vi "Line Prototype 1.2.vi"() -> ()   [LabVIEW 2009]
uses:
  <vilib>/vision/Image Controls.llb/IMAQ Image.ctl
  <vilib>/Analysis/3filter.llb/Filter Passband Type.ctl
  <vilib>/Analysis/3filter.llb/Butterworth Filter (DBL).vi
  <vilib>/vision/NI_Vision_Development_Module.lvlib
  <vilib>/Analysis/NI_AALBase.lvlib
panel:
  in  "low  2":dbl=0.12500000000000006 format="%0.4f"
  in  "high 2":dbl=60.0 format="%0.2f"
  in  "sampling 2":dbl=1.0 format="%0.2f"
  out "LED BLUE":bool
  out "Waveform RED 2":dbl[](graph)
  in  "playtime":dbl=10.0
  out "Frame Number":i32
  in  "Frame Start":i32=2100
  out "LED RED":bool
  in  "low":dbl=0.12500000000000006 format="%0.4f"
  out "Waveform RED":dbl[](graph)
  in  "high":dbl=60.0 format="%0.2f"
  in  "sampling":dbl=1.0 format="%0.2f"
  out "Image Out 2":T1
  out "Line Profile  BLUE":cluster{"x0":sgl, "dx":sgl, "Pixels Line":sgl[]}(graph) caption="Line Profile"
  out "Line Profile RED":cluster{"x0":sgl, "dx":sgl, "Pixels Line":sgl[]}(graph) caption="Line Profile"
  out "Image Out":T1
  out "Green ROI":T1(plugin-control)
  out "Image":T1(plugin-control)
  in  "stop":bool
  in  "AVI Path":path
  # "BLUE"
  # "RED"
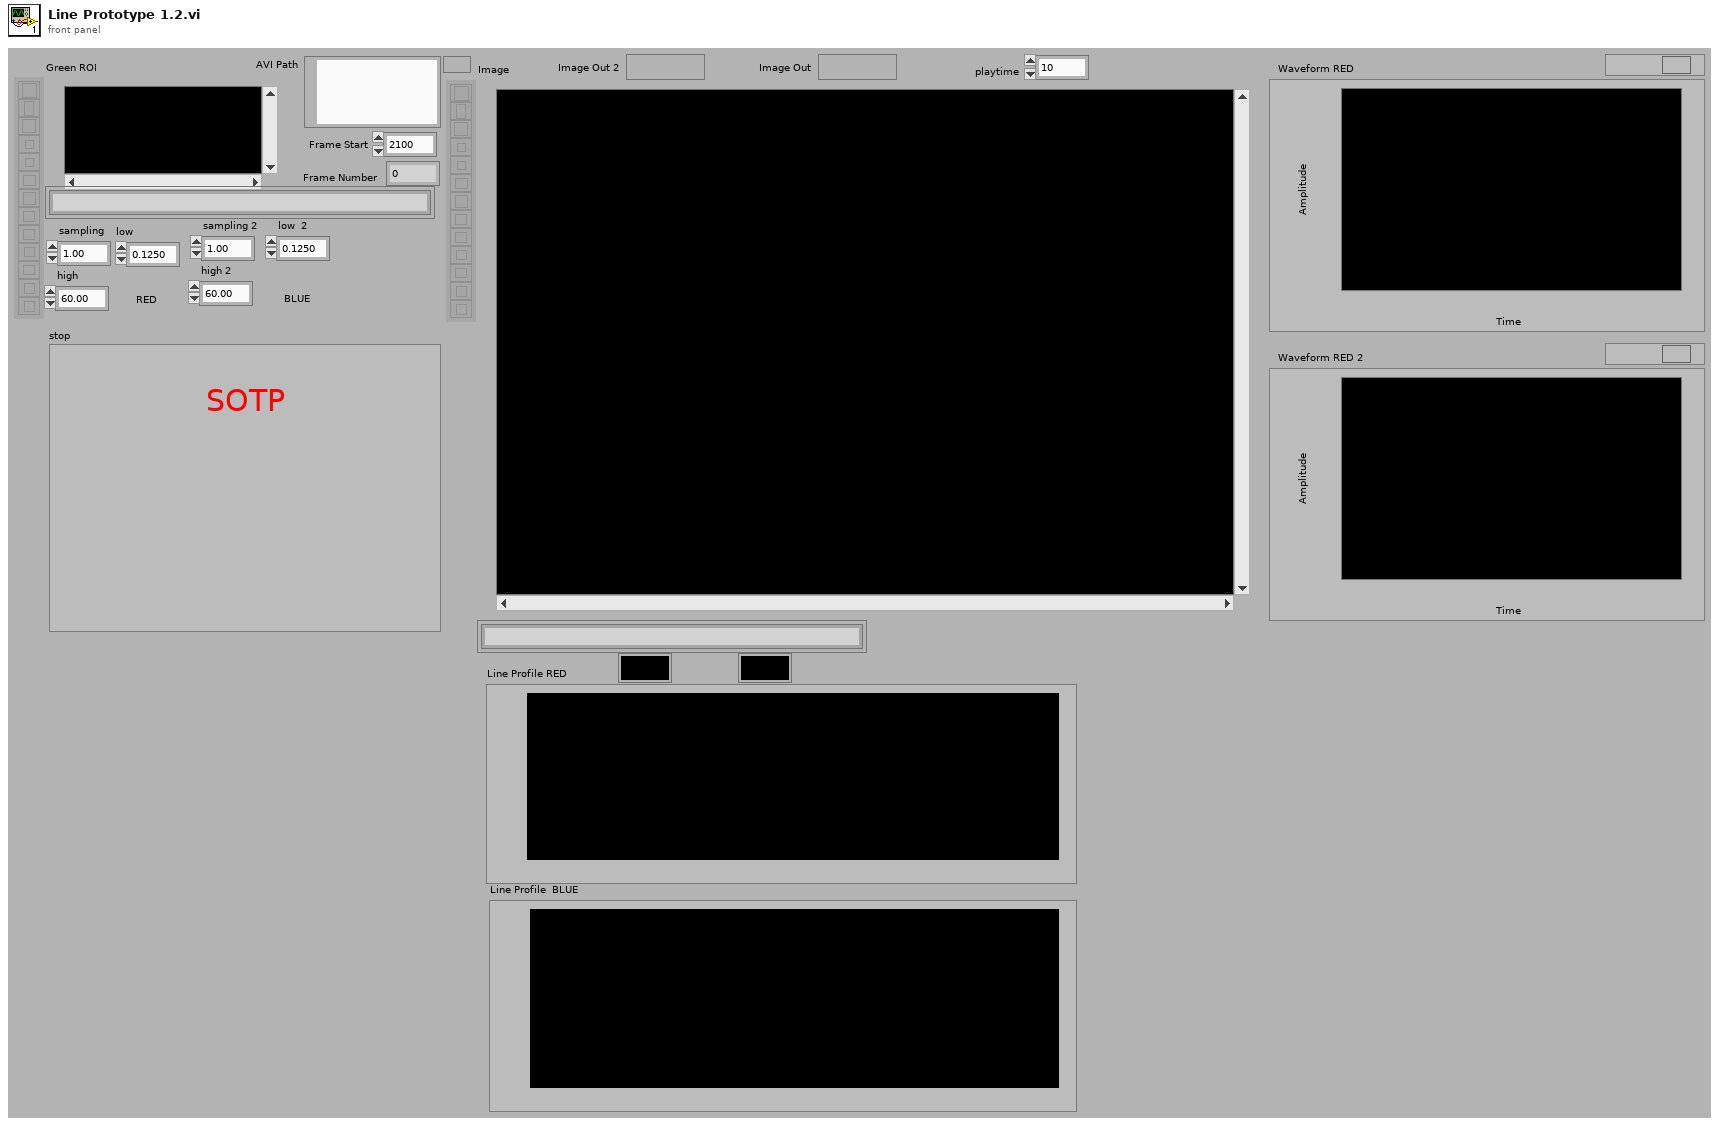
[diagram p1: front panel]
types:
  T1 = typedef "IMAQ Image.ctl" = refnum<image>
  T2 = typedef "NI_AALBase.lvlib/Filter Passband Type.ctl" = enum32{"Lowpass", "Highpass", "Bandpass", "Bandstop"}
  T3 = cluster{"Left":i32, "Top":i32, "Right":i32, "Bottom":i32}
  T4 = cluster{"Global Rectangle":i32[], "Contours":cluster{"ID":enum32{"External", "Internal"}, "Type":u32, "Coordinates":i32[]}[]}
  T5 = cluster{"ID":enum32{"External", "Internal"}, "Type":u32, "Coordinates":i32[]}[]
  T6 = cluster{"ID":enum32{"External", "Internal"}, "Type":u32, "Coordinates":i32[]}
  T7 = cluster{"Min":sgl, "Max":sgl, "Mean":sgl, "Std Dev":sgl, "Count":i32}
  T8 = typedef "AviRefnum.ctl" = refnum<k1>
  T9 = typedef "Image Type" = u32
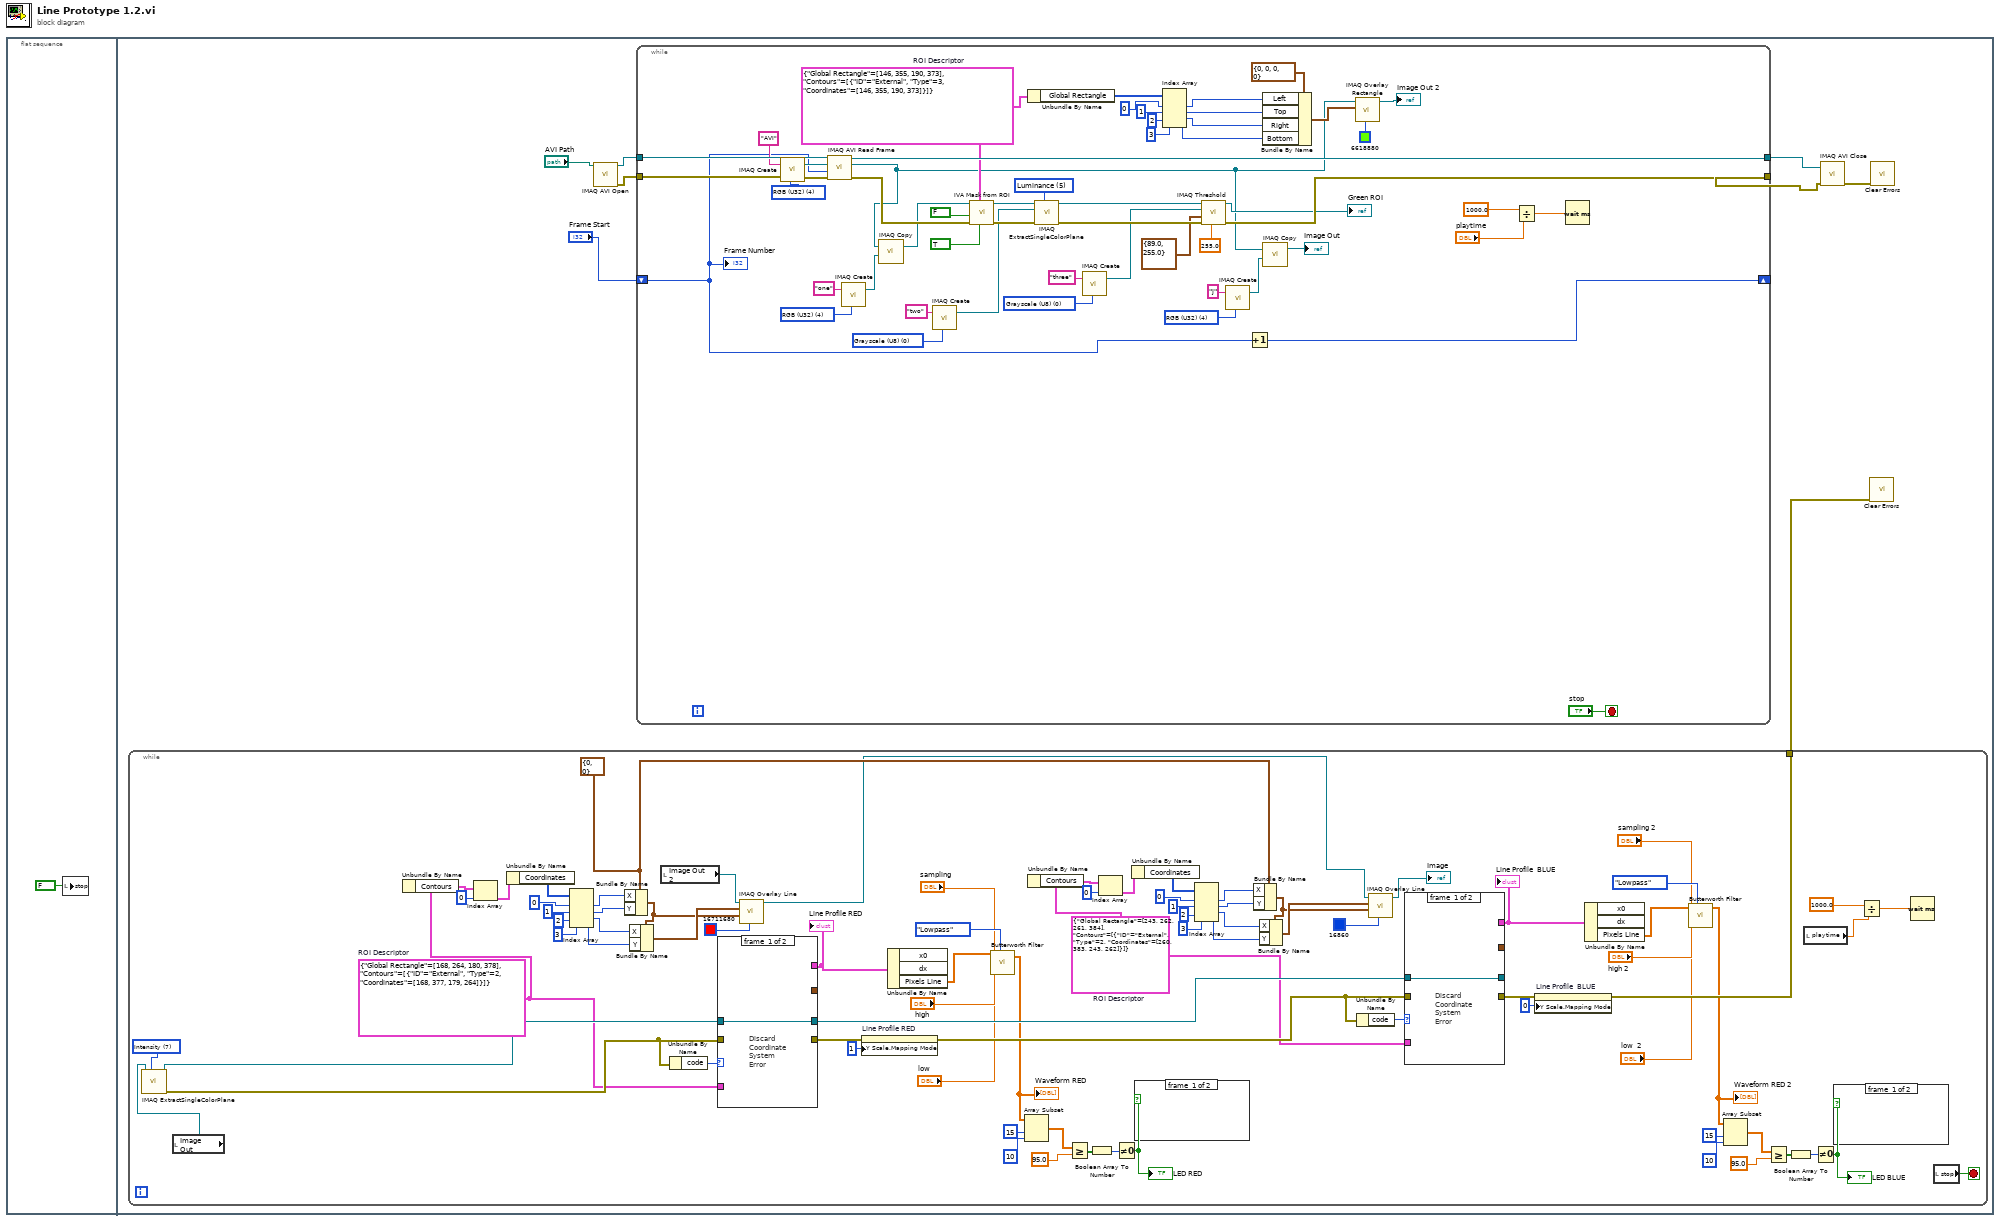
[diagram p0: block diagram]
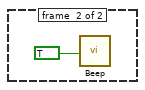
[diagram p2: hidden frame]
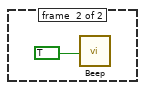
[diagram p3: hidden frame]
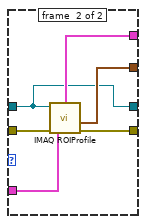
[diagram p4: hidden frame]
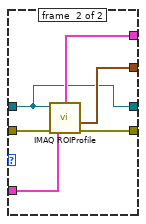
[diagram p5: hidden frame]
diagram:
  n1 = flat-sequence {
    frame #0 {
      n2 = local write "stop"(FALSE ("stop")) -> ()
    }
    frame #1 {
      n3 = while {
        tunnel: [w77] -> w2
        stop <- w78 stop-if-true
        w45 = cluster{"X":i32, "Y":i32} {"X"=0, "Y"=0} ("End Point")
        w48 = T4 {"Global Rectangle"=[243, 262, 261, 384], "Contours"=[{"ID"=enum."External", "Type"=2, "Coordinates"=[260, 383, 243, 262]}]}  # ROI Descriptor
        w68 = T4 {"Global Rectangle"=[168, 264, 180, 378], "Contours"=[{"ID"=enum."External", "Type"=2, "Coordinates"=[168, 377, 179, 264]}]}  # ROI Descriptor
        w90 = 7 items=["Red", "Green", "Blue", "Hue", "Saturation", "Luminance", "Value", "Intensity"] ("Color Plane")
        n4 = local read "Image Out"() -> (w79:T1)
        n5 = call "IMAQ ExtractSingleColorPlane"("Color Plane"=w90, "Image Src"=w79) -> ("error out"=w89:errorcluster, "Image Dst Out"=w85:T1)  [unwired: 2 in, 6 out]
        n6 = Unbundle By Name(w68) -> ("Contours"=w65:T5)
        n7 = Index Array(array=w65, index=0) -> (element=w63:T6)
        n8 = Unbundle By Name(w63) -> ("Coordinates"=w62:i32[])
        n9 = Index Array(array=w62, index #1=0 ("index"), index #2=1 ("index"), index #3=2 ("index"), index #4=3 ("index")) -> (element #1=w72:i32, element #2=w71:i32, element #3=w70:i32, element #4=w69:i32)
        n10 = Bundle By Name(cluster=w45, "X"=w72, "Y"=w71) -> (w46:cluster{"X":i32, "Y":i32})
        n11 = Bundle By Name(cluster=w46, "X"=w70, "Y"=w69) -> (w47:cluster{"X":i32, "Y":i32})
        n12 = local read "Image Out 2"() -> (w67:T1)
        n13 = Unbundle By Name(w89) -> ("code"=w84:i32)
        n14 = case shown="Default" w84 {
          tunnel: w89 -> [_ w106]
          tunnel: [_ w105] -> _
          tunnel: [_ w104] -> w87
          tunnel: w85 -> [w100 w101]
          tunnel: [_ w103] -> w39
          tunnel: w68 -> [_ w102]
          tunnel: [w100 w101] -> w81
          frame #0 {
            # "Discard\nCoordinate\nSystem\nError"
          }
          frame #1 {
            n15 = call "IMAQ ROIProfile"("error in (no error)"=w106, "ROI Descriptor"=w102, "Image"=w101) -> ("ROI Pixel Statistics"=w105:T7, "error out"=w104:errorcluster, "ROI Graph"=w103:cluster{"x0":sgl, "dx":sgl, "Pixels Line":sgl[]})  [unwired: 3 out]
          }
        }
        "Line Profile RED" <- w39
        n16 = call "IMAQ Overlay Line"("Color"=u32 16711680, "End Point"=w46, "Start Point"=w47, "Image"=w67) -> ("Image Out"=w42:T1)  [unwired: 6 in, 1 out]
        n17 = property on="Line Profile RED" class="WFGraph"(error in=w87, "Y Scale.Mapping Mode"=u8 1) -> (error out=w86:errorcluster)  [unwired: 1 in, 1 out]
        n18 = Unbundle By Name(w39) -> ("Pixels Line"=w38:sgl[])  [unwired: 2 out]
        n19 = call-poly <vilib>:"Butterworth Filter.vi"("filter type"=Filter_Passband_Type."Lowpass", "low cutoff freq: fl"="low", "high cutoff freq: fh"="high", "sampling freq: fs"="sampling", "X"=w38) -> ("Filtered X"=w34:dbl[])  [unwired: 3 in, 1 out]
        "Waveform RED" <- w34
        n20 = Array Subset(array=w34, index=15, length=10) -> (w31:dbl[])
        n21 = Unbundle By Name(w48) -> ("Contours"=w58:T5)
        n22 = Greater Or Equal?(x=w31, y=95.0) -> (x >= y?=w29:bool[])
        n23 = Boolean Array To Number(Boolean array=w29) -> (number=w26:u32)
        n24 = Index Array(array=w58, index=0) -> (element=w60:T6)
        n25 = Not Equal To 0?(x=w26) -> (x != 0?=w24:bool)
        "LED RED" <- w24
        n26 = Unbundle By Name(w60) -> ("Coordinates"=w61:i32[])
        n27 = case shown="True" w24 {
          frame #0 {
          }
          frame #1 {
            n28 = call <vilib>:"Beep.vi"("use system alert? (T)"=TRUE) -> ()  [unwired: 11 in]
          }
        }
        n29 = Index Array(array=w61, index #1=0 ("index"), index #2=1 ("index"), index #3=2 ("index"), index #4=3 ("index")) -> (element #1=w53:i32, element #2=w54:i32, element #3=w55:i32, element #4=w56:i32)
        n30 = Bundle By Name(cluster=w45, "X"=w53, "Y"=w54) -> (w43:cluster{"X":i32, "Y":i32})
        n31 = Bundle By Name(cluster=w43, "X"=w55, "Y"=w56) -> (w44:cluster{"X":i32, "Y":i32})
        n32 = Unbundle By Name(w86) -> ("code"=w80:i32)
        n33 = call "IMAQ Overlay Line"("Color"=u32 16860, "End Point"=w43, "Start Point"=w44, "Image"=w42) -> ("Image Out"=→"Image":T1)  [unwired: 6 in, 1 out]
        n34 = case shown="Default" w80 {
          tunnel: w86 -> [_ w99]
          tunnel: [_ w98] -> _
          tunnel: [_ w97] -> w82
          tunnel: w81 -> [w93 w94]
          tunnel: [_ w96] -> w12
          tunnel: w48 -> [_ w95]
          tunnel: [w93 w94] -> _
          frame #0 {
            # "Discard\nCoordinate\nSystem\nError"
          }
          frame #1 {
            n35 = call "IMAQ ROIProfile"("error in (no error)"=w99, "ROI Descriptor"=w95, "Image"=w94) -> ("ROI Pixel Statistics"=w98:T7, "error out"=w97:errorcluster, "ROI Graph"=w96:cluster{"x0":sgl, "dx":sgl, "Pixels Line":sgl[]})  [unwired: 3 out]
          }
        }
        "Line Profile  BLUE" <- w12
        n36 = property on="Line Profile  BLUE" class="WFGraph"(error in=w82, "Y Scale.Mapping Mode"=u8 0) -> (error out=w77:errorcluster)  [unwired: 1 in, 1 out]
        n37 = Unbundle By Name(w12) -> ("Pixels Line"=w15:sgl[])  [unwired: 2 out]
        n38 = call-poly <vilib>:"Butterworth Filter.vi"("filter type"=Filter_Passband_Type."Lowpass", "low cutoff freq: fl"="low  2", "high cutoff freq: fh"="high 2", "sampling freq: fs"="sampling 2", "X"=w15) -> ("Filtered X"=w11:dbl[])  [unwired: 3 in, 1 out]
        "Waveform RED 2" <- w11
        n39 = Array Subset(array=w11, index=15, length=10) -> (w21:dbl[])
        n40 = Greater Or Equal?(x=w21, y=95.0) -> (x >= y?=w19:bool[])
        n41 = Boolean Array To Number(Boolean array=w19) -> (number=w18:u32)
        n42 = local read "playtime"() -> (w25:dbl)
        n43 = Not Equal To 0?(x=w18) -> (x != 0?=w17:bool)
        "LED BLUE" <- w17
        n44 = case shown="True" w17 {
          frame #0 {
          }
          frame #1 {
            n45 = call <vilib>:"Beep.vi"("use system alert? (T)"=TRUE) -> ()  [unwired: 11 in]
          }
        }
        n46 = Divide(x=1000.0, y=w25) -> (x/y=w28:dbl)
        n47 = Wait (ms)(milliseconds to wait=w28) -> ()  [unwired: 1 out]
        n48 = local read "stop"() -> (w78:bool)
      }
      n49 = call "IMAQ AVI Open"("AVI Path"="AVI Path") -> ("error out"=w4:errorcluster, "Avi Refnum"=w5:T8)  [unwired: 9 in]
      n50 = while {
        tunnel: w5 -> [w157]
        tunnel: w4 -> [w160]
        tunnel: [w148] -> w6
        tunnel: [w154] -> w7
        shift-right: [w143] -> _
        shift-left: "Frame Start" -> [w142]
        stop <- "stop" stop-if-true
        w112 = T9 4 items=["Grayscale (U8)", "Grayscale (I16)", "Grayscale (SGL)", "Complex (CSG)", "RGB (U32)", "HSL (U32)", "RGB (U64)", "Grayscale (U16)"] ("Image Type")
        w118 = T9 0 items=["Grayscale (U8)", "Grayscale (I16)", "Grayscale (SGL)", "Complex (CSG)", "RGB (U32)", "HSL (U32)", "RGB (U64)", "Grayscale (U16)"] ("Image Type")
        w124 = 5 items=["Red", "Green", "Blue", "Hue", "Saturation", "Luminance", "Value", "Intensity"] ("Color Plane")
        w144 = T9 0 items=["Grayscale (U8)", "Grayscale (I16)", "Grayscale (SGL)", "Complex (CSG)", "RGB (U32)", "HSL (U32)", "RGB (U64)", "Grayscale (U16)"] ("Image Type")
        w145 = T9 4 items=["Grayscale (U8)", "Grayscale (I16)", "Grayscale (SGL)", "Complex (CSG)", "RGB (U32)", "HSL (U32)", "RGB (U64)", "Grayscale (U16)"] ("Image Type")
        w141 = T4 {"Global Rectangle"=[146, 355, 190, 373], "Contours"=[{"ID"=enum."External", "Type"=3, "Coordinates"=[146, 355, 190, 373]}]}  # ROI Descriptor
        w155 = T9 4 items=["Grayscale (U8)", "Grayscale (I16)", "Grayscale (SGL)", "Complex (CSG)", "RGB (U32)", "HSL (U32)", "RGB (U64)", "Grayscale (U16)"] ("Image Type")
        n51 = call "IMAQ Create"("Image Name"="AVI", "Image Type"=w155, "error in (no error)"=w160) -> ("New Image"=w158:T1, "error out"=w159:errorcluster)  [unwired: 2 in]
        n52 = call "IMAQ AVI Read Frame"("error in (no error)"=w159, "Frame Number"=w142, "Image"=w158, "Avi Refnum"=w157) -> ("error out"=w149:errorcluster, "Image Out"=w109:T1, "Avi Refnum (duplicate)"=w154:T8)  [unwired: 4 in, 1 out]
        n53 = call "IMAQ Create"("Image Name"="one", "Image Type"=w145) -> ("New Image"=w147:T1)  [unwired: 3 in, 1 out]
        n54 = call "IMAQ Copy"("Image Dst"=w147, "Image Src"=w109) -> ("Image Dst Out"=w128:T1)  [unwired: 4 in, 1 out]
        n55 = call "IMAQ Create"("Image Name"="two", "Image Type"=w144) -> ("New Image"=w114:T1)  [unwired: 3 in, 1 out]
        n56 = call <vilib>:"IVA Mask from ROI.vi"("Shrink"=TRUE, "ROI Descriptor"=w141, "error in (no error)"=w149, "Out / In"=FALSE, "Image Src"=w128) -> ("error out"=w126:errorcluster, "Image Out"=w123:T1)  [unwired: 5 out]
        n57 = Unbundle By Name(w141) -> ("Global Rectangle"=w137:i32[])
        n58 = call "IMAQ ExtractSingleColorPlane"("Color Plane"=w124, "error in (no error)"=w126, "Image Dst"=w114, "Image Src"=w123) -> ("error out"=w122:errorcluster, "Image Dst Out"=w120:T1)  [unwired: 6 out]
        n59 = call "IMAQ Create"("Image Name"="three", "Image Type"=w118) -> ("New Image"=w116:T1)  [unwired: 3 in, 1 out]
        n60 = Index Array(array=w137, index #1=0 ("index"), index #2=1 ("index"), index #3=2 ("index"), index #4=3 ("index")) -> (element #1=w136:i32, element #2=w135:i32, element #3=w134:i32, element #4=w133:i32)
        n61 = call "IMAQ Threshold"("Replace Value"=sgl 255.0, "error in (no error)"=w122, "Range"=cluster{"Lower value":sgl, "Upper value":sgl} {"Lower value"=89.0, "Upper value"=255.0}, "Image Dst"=w116, "Image Src"=w120) -> ("error out"=w148:errorcluster, "Image Dst Out"=→"Green ROI":T1)  [unwired: 1 in, 4 out]
        n62 = call "IMAQ Create"("Image Name"="j", "Image Type"=w112) -> ("New Image"=w110:T1)  [unwired: 3 in, 1 out]
        n63 = Increment(x=w142) -> (x+1=w143:i32)
        n64 = Bundle By Name(cluster=T3 {"Left"=0, "Top"=0, "Right"=0, "Bottom"=0} ("Rectangle"), "Left"=w136, "Top"=w135, "Right"=w134, "Bottom"=w133) -> (w139:T3)
        n65 = call "IMAQ Copy"("Image Dst"=w110, "Image Src"=w109) -> ("Image Dst Out"=→"Image Out":T1)  [unwired: 4 in, 1 out]
        n66 = call "IMAQ Overlay Rectangle"("Color"=u32 6618880, "Rectangle"=w139, "Image"=w109) -> ("Image Out"=→"Image Out 2":T1)  [unwired: 7 in, 1 out]
        n67 = Divide(x=1000.0, y="playtime") -> (x/y=w152:dbl)
        n68 = Wait (ms)(milliseconds to wait=w152) -> ()  [unwired: 1 out]
        "Frame Number" <- w142
      }
      n69 = call "IMAQ AVI Close"("error in (no error)"=w6, "Avi Refnum"=w7) -> ("error out"=w8:errorcluster)  [unwired: 9 in]
      n70 = call <vilib>:"Clear Errors.vi"("error in (no error)"=w2) -> ()  [unwired: 6 in, 1 out]
      n71 = call <vilib>:"Clear Errors.vi"("error in (no error)"=w8) -> ()  [unwired: 6 in, 1 out]
    }
  }
